vi "Request Elements 2.vi"(8 "error in (no error)":errorcluster, 11 "Event Response Handler in":refnum<class "Event Response Handler.lvclass">) -> (0 "error out":errorcluster, 3 "Event Response Handler out":refnum<class "Event Response Handler.lvclass">)   [LabVIEW 2020, in "Event Response Handler.lvclass"]
uses:
  Event Response Handler.lvclass
  Event Response Handler.lvclass/Event Response Handler.ctl
  ElementsValue/ElementsValue.lvclass
  ElementsValue/Some Fancy Data.ctl
panel:
  out "Value":T1
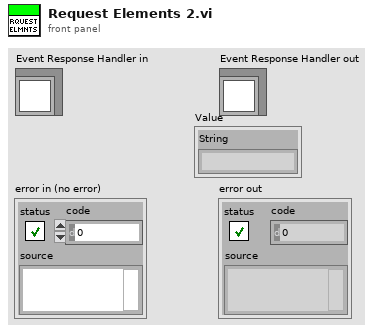
[diagram p1: front panel]
types:
  T1 = typedef "Futures-Examples.lvlib/ElementsValue.lvclass/Some Fancy Data.ctl" = cluster{"String":string}
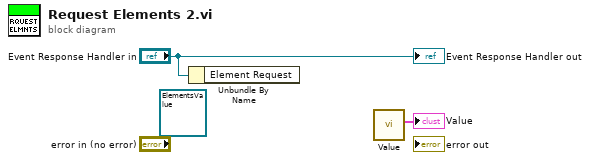
[diagram p0: block diagram]
diagram:
  (unwired) refnum<class "ElementsValue.lvclass"> refnum ("Futures-Examples.lvlib:ElementsValue.lvclass")
  n1 = Unbundle By Name("Event Response Handler in") -> ()  [unwired: 1 out]
  n2 = call "Value.vi"() -> ("Value"=→"Value":T1)  [unwired: 11 in]
  "Event Response Handler out" <- "Event Response Handler in"
